vi "TotalTime.vi"(3 "factor":i32=1, 4 "loadTime":i32, 5 "preloadTime":i32) -> (0 "strSec":string, 1 "strHour":string, 2 "total":i32)   [LabVIEW 2015]
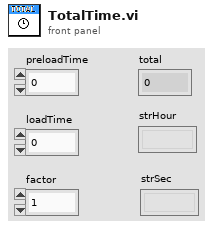
[diagram p1: front panel]
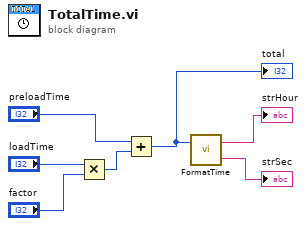
[diagram p0: block diagram]
diagram:
  n1 = Multiply(x="loadTime", y="factor") -> (x*y=w4:i32)
  n2 = Add(x="preloadTime", y=w4) -> (x+y=w5:i32)
  "total" <- w5
  n3 = call "FormatTime.vi"("secondNum"=w5) -> ("secondText"=→"strSec":string, "timeText"=→"strHour":string)  [unwired: 1 in]
